vi "Multichannel Recording0.1.vi"() -> ()   [LabVIEW 2014]
uses:
  Timed Recorder Project/Single Channel Volt Recording Folder/Enum State Typedef.ctl
  <vilib>/Utility/error.llb/DialogType.ctl
  <vilib>/_DAQmxBase/Internals/DAQmxBase Create Channel (AI-Voltage-Basic).vi
  <vilib>/_DAQmxBase/Internals/DAQmxBase Timing (Sample Clock).vi
  <vilib>/_DAQmxBase/Internals/DAQmxBase Read (Analog 2D DBL NChan NSamp).vi
panel:
  in  "Tab Control":T1(tab)
  in  "Use Channel 0":bool caption="In Use?"
  in  "Amplifier Channel 0":T2 {"Amplifier Model" items=["Select a Model", "AM 1700", "BMA 200"]}
  out "Channel 0 Chart":waveform(dbl)(graph)
  in  "User Data Channel 0":T3
  in  "Use Channel 1":bool caption="In Use?"
  out "Channel 1 Chart":waveform(dbl)(graph)
  in  "User Data Channel 1":T3
  in  "Amplifier Channel 1":T2 {"Amplifier Model" items=["Select a Model", "AM 1700", "BMA 200"]}
  in  "Use Channel 2":bool caption="In Use?"
  out "Channel 2 Chart":waveform(dbl)(graph)
  in  "User Data Channel 2":T3
  in  "Amplifier Channel 2":T2 {"Amplifier Model" items=["Select a Model", "AM 1700", "BMA 200"]}
  in  "Use Channel 3":bool caption="In Use?"
  out "Channel 3 Chart":waveform(dbl)(graph)
  in  "User Data Channel 3":T3
  in  "Amplifier Channel 3":T2 {"Amplifier Model" items=["Select a Model", "AM 1700", "BMA 200"]}
  out "Overview Chart":waveform(dbl)[](graph)
  in  "Stop Preview":bool
  in  "OK Button":bool
  out "State":T4
  in  "Clear Display":bool
  in  "Preview Button":bool
  out "Iterations Recorded":i32
  in  "Recording Time (seconds)":dbl
  in  "Sample Rate":i32=1000
  in  "Stop Button":bool
  out "Start Time hr/min":string
  out "Date mm/dd/yy":string
  in  "Exit Button":bool
  in  "Record Button":bool
  # "MSU EFISH Lab Single Channel Electronic Pulse Recorder"
  # "Must enter numbers into here before you start"
  # "Blue for On\nOrange for Off"
  # "DC"
  # "AC"
  # "Blue for AC and Orange for DC"
  # "Blue for On\nOrange for Off"
  # "DC"
  # "AC"
  # "Blue for AC and Orange for DC"
  # "Blue for On\nOrange for Off"
  # "DC"
  # "AC"
  # "Blue for AC and Orange for DC"
  # "Blue for On\nOrange for Off"
  # "DC"
  # "AC"
  # "Blue for AC and Orange for DC"
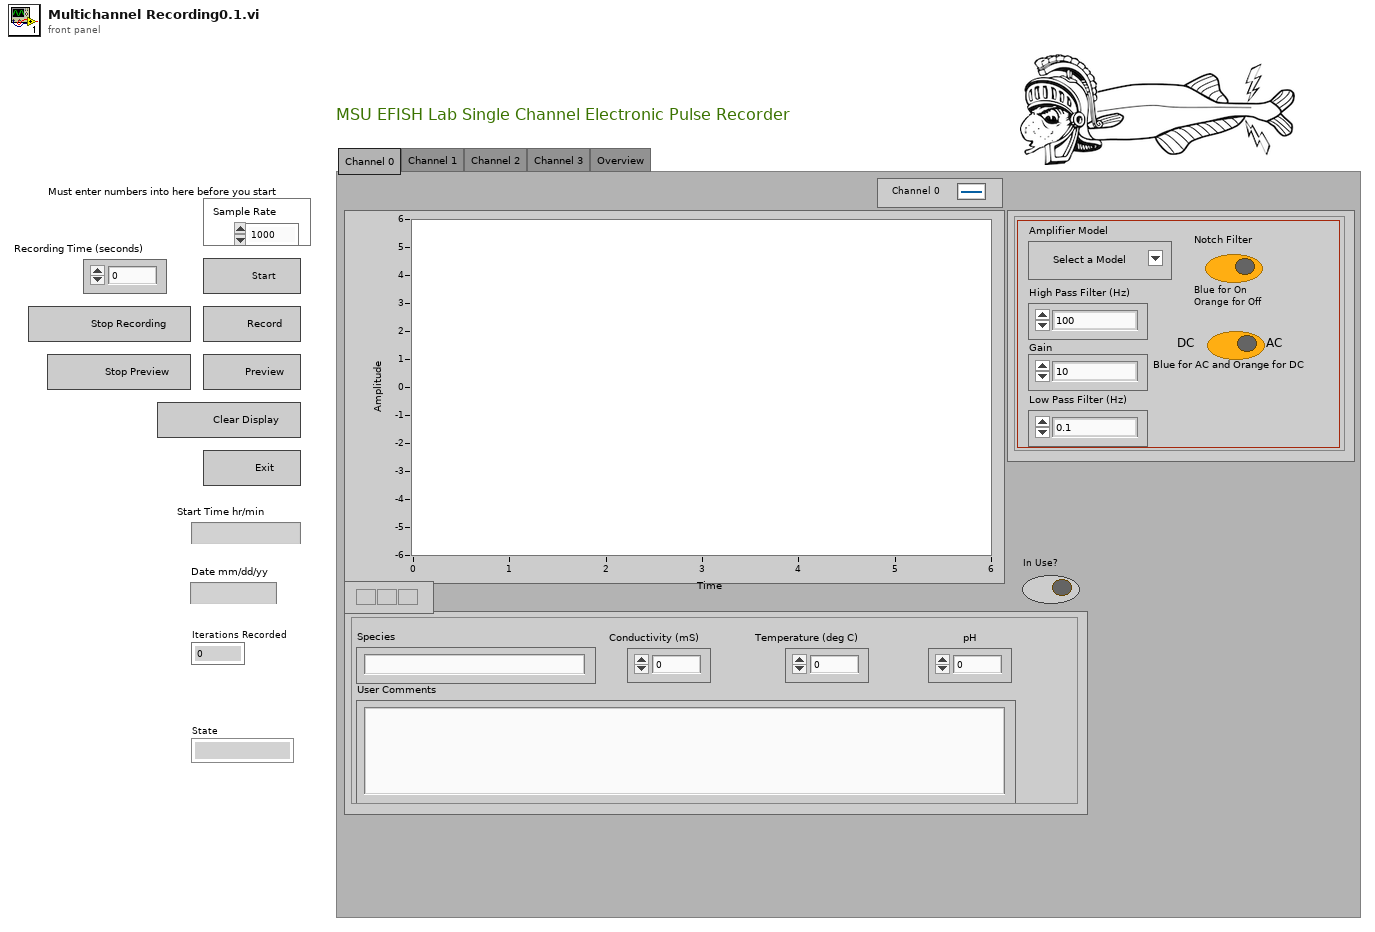
[diagram p1: front panel]
types:
  T1 = enum32{"Channel 0", "Channel 1", "Channel 2", "Channel 3", "Overview"}
  T2 = cluster{"Low Pass Filter (Hz)":enum16{"0.1", "1", "3", "10", "30", "100", "300"}, "Gain ":enum16{"10", "20", "50", "100", "200", "500", "1000", "2k", "5k", "10k", "20k", "50k"}, "High Pass Filter (Hz)":enum16{"100", "500", "1000", "3000", "5000", "10,000", "20,000", "30,000", "50,000"}, "Notch Filter":bool, "Amplifier Model":u16, "AC/DC Switch":bool}
  T3 = cluster{"pH":dbl, "Conductivity (mS)":dbl, "Temperature (deg C)":dbl, "User Comments":string, "Species":string}
  T4 = typedef "Enum State Typedef.ctl" = enum16{"", "Beginning State", "Set the Sample Clock", "Prepreview Handling", "Clear Display", "Preview Data", "Stop", "Exit", "Record", "Create File"}
  T5 = enum16{"open", "open or create", "create or replace", "create", "open (read-only)"}
  T6 = typedef "DialogType.ctl" = u16
  T7 = cluster{"data":dbl[][], dbl[][], i32, i32, dbl, "Use Channel 2":bool}
  T8 = cluster{"data":dbl[][], dbl[][], i32, i32, dbl, "Use Channel 1":bool}
  T9 = cluster{"data":dbl[][], dbl[][], i32, i32, dbl, "Use Channel 0":bool}
  T10 = cluster{"data":dbl[][], dbl[][], i32, i32, dbl, "Use Channel 3":bool}
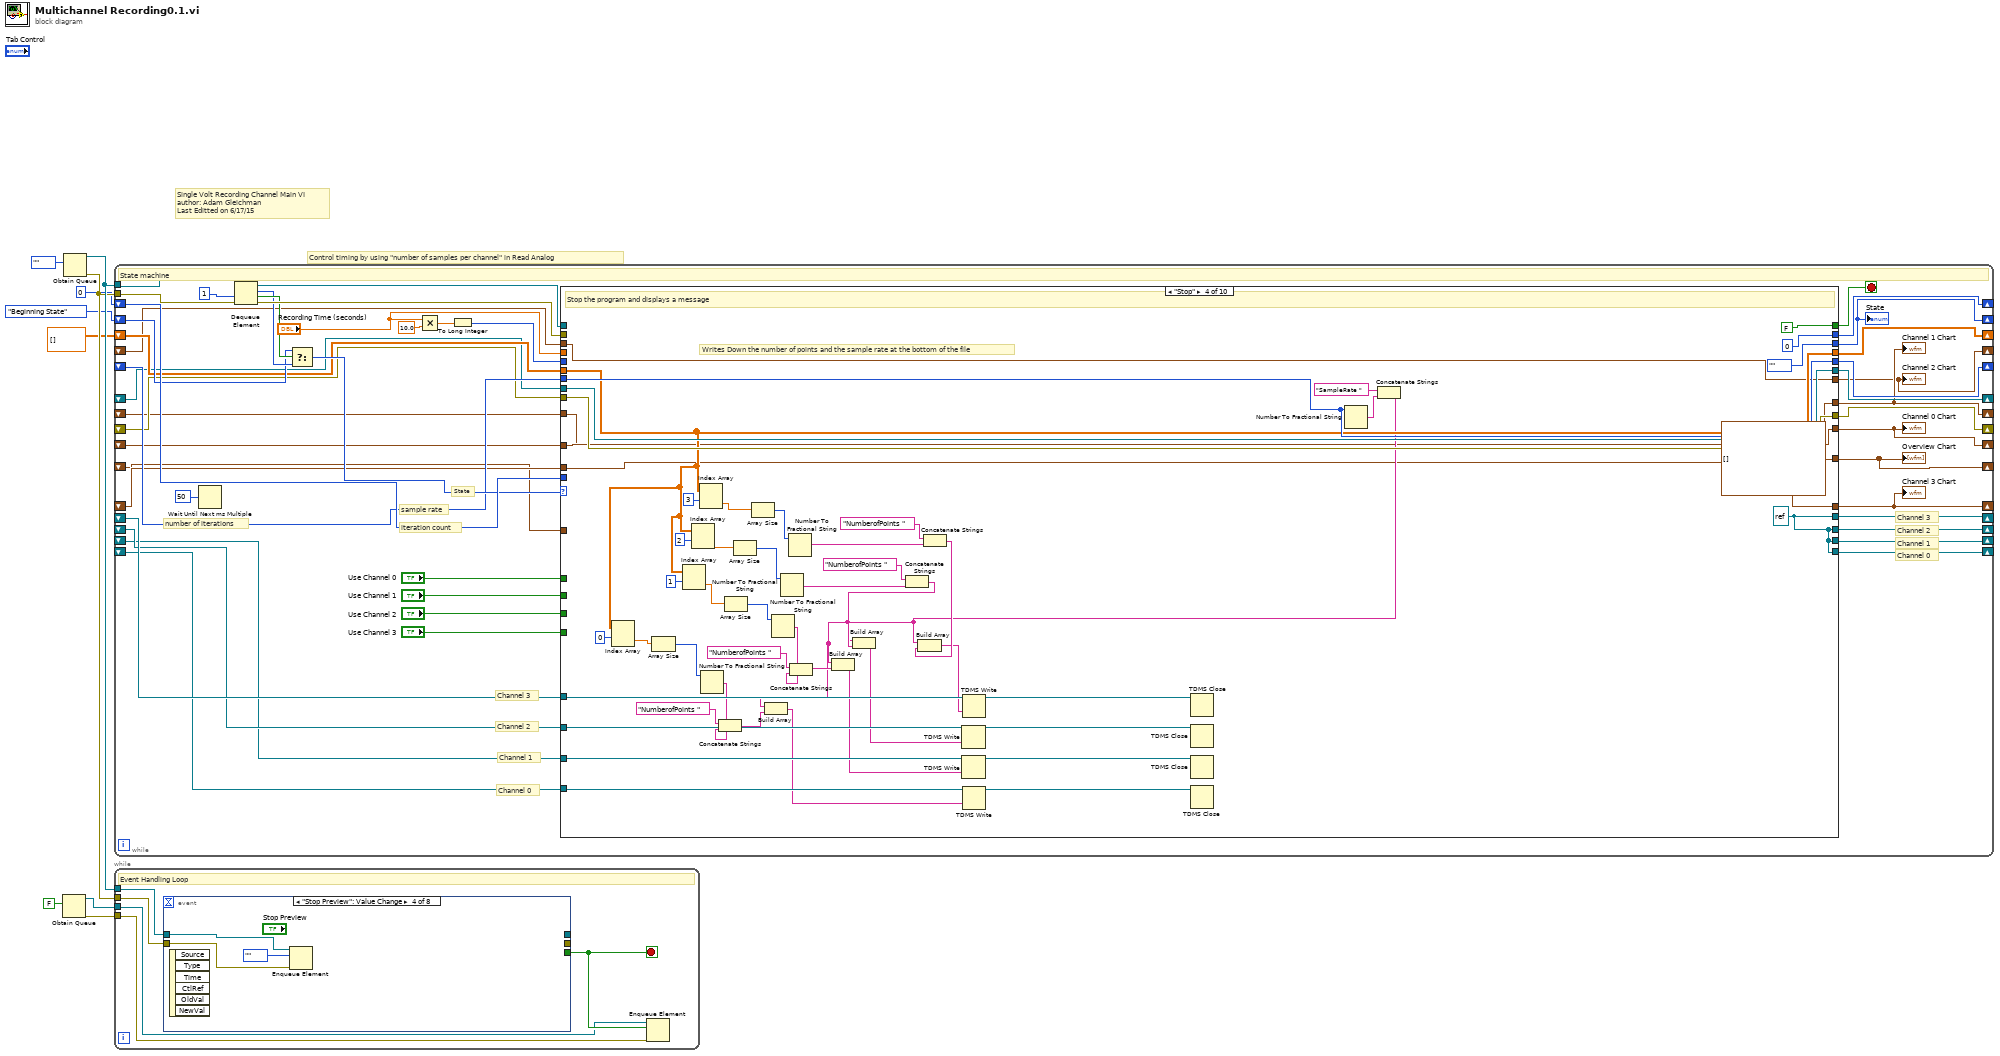
[diagram p0: block diagram]
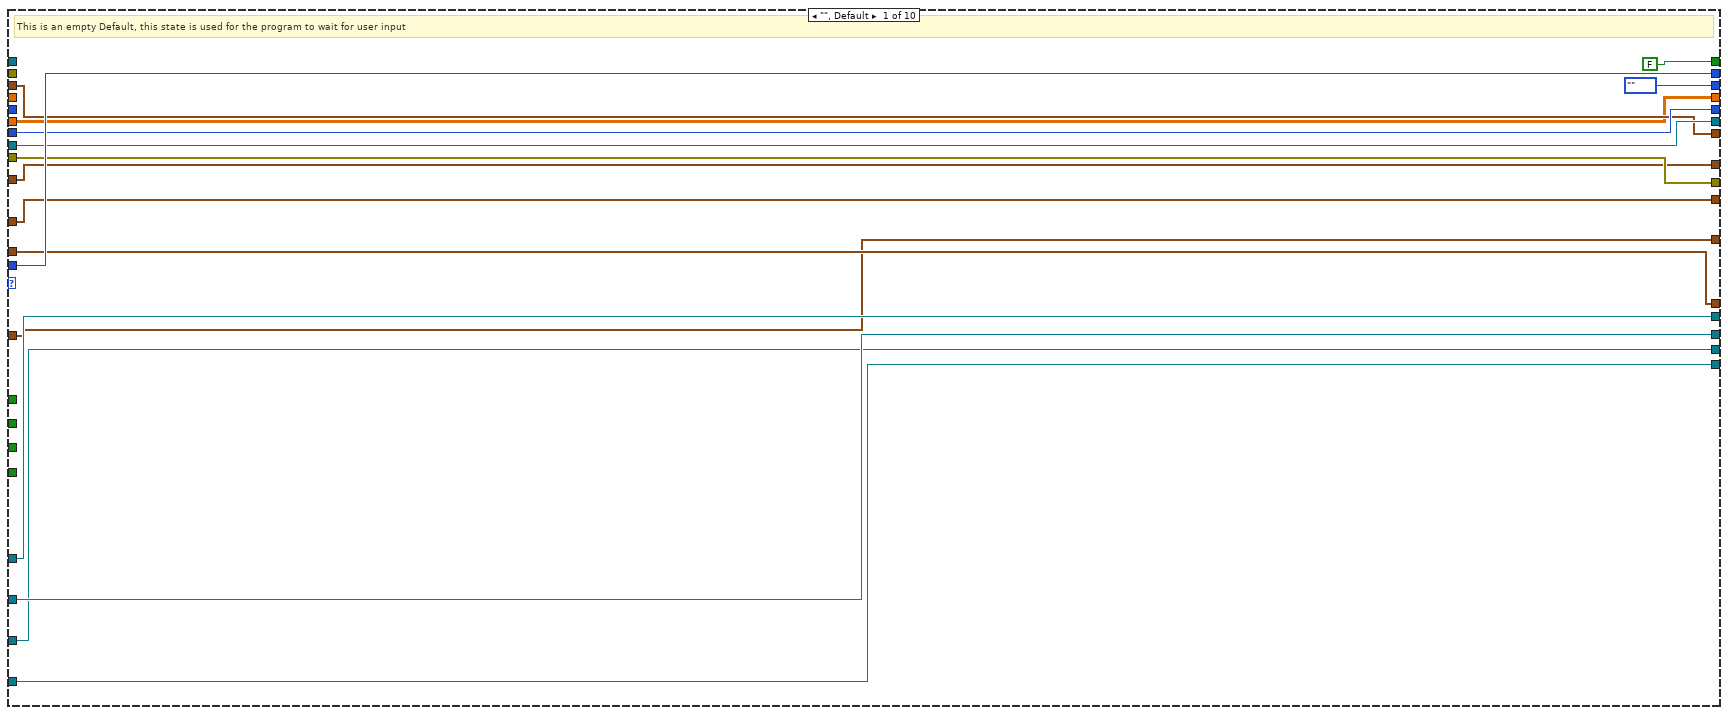
[diagram p2: hidden frame]
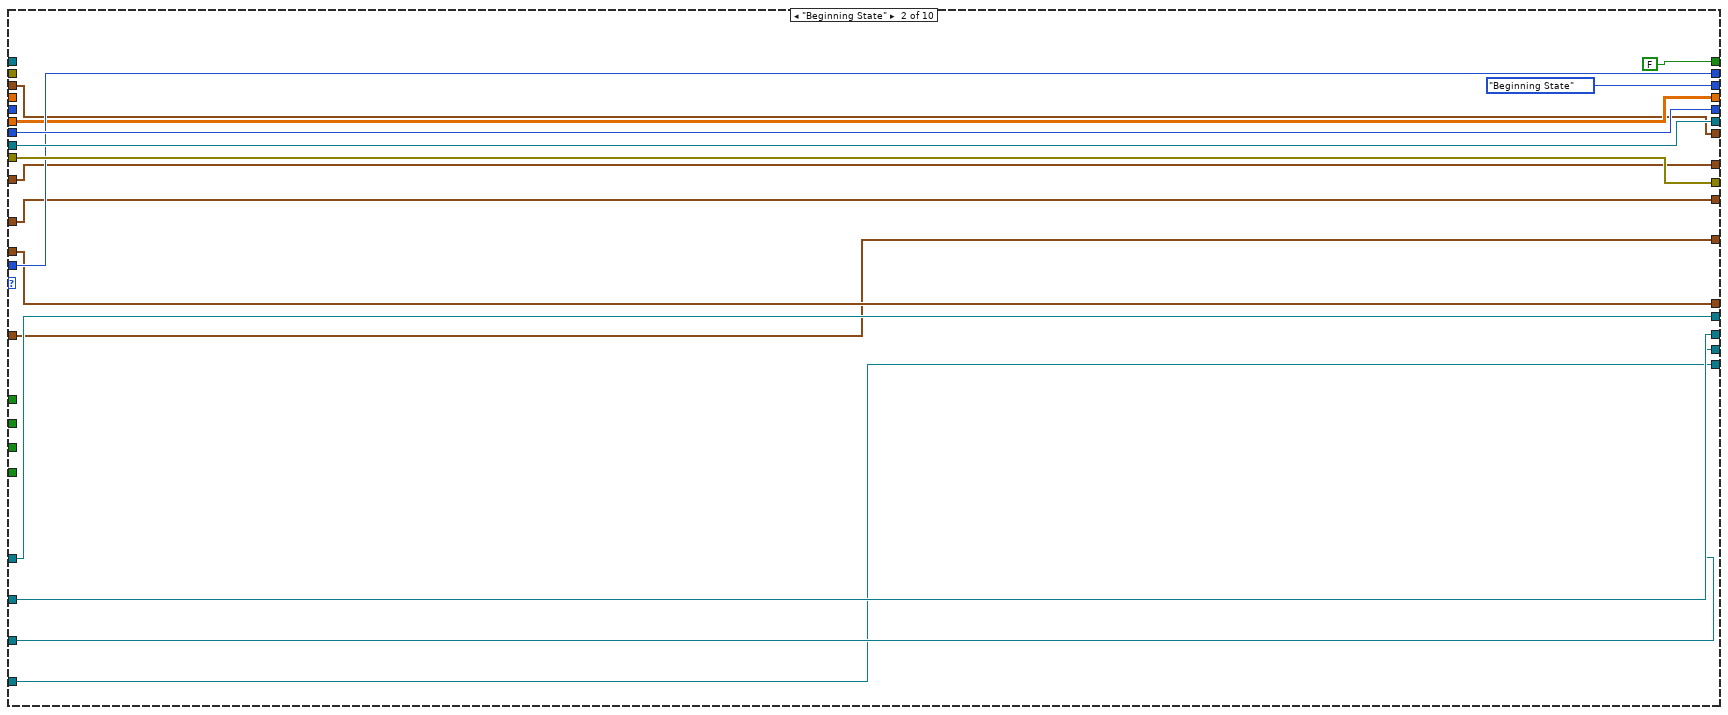
[diagram p3: hidden frame]
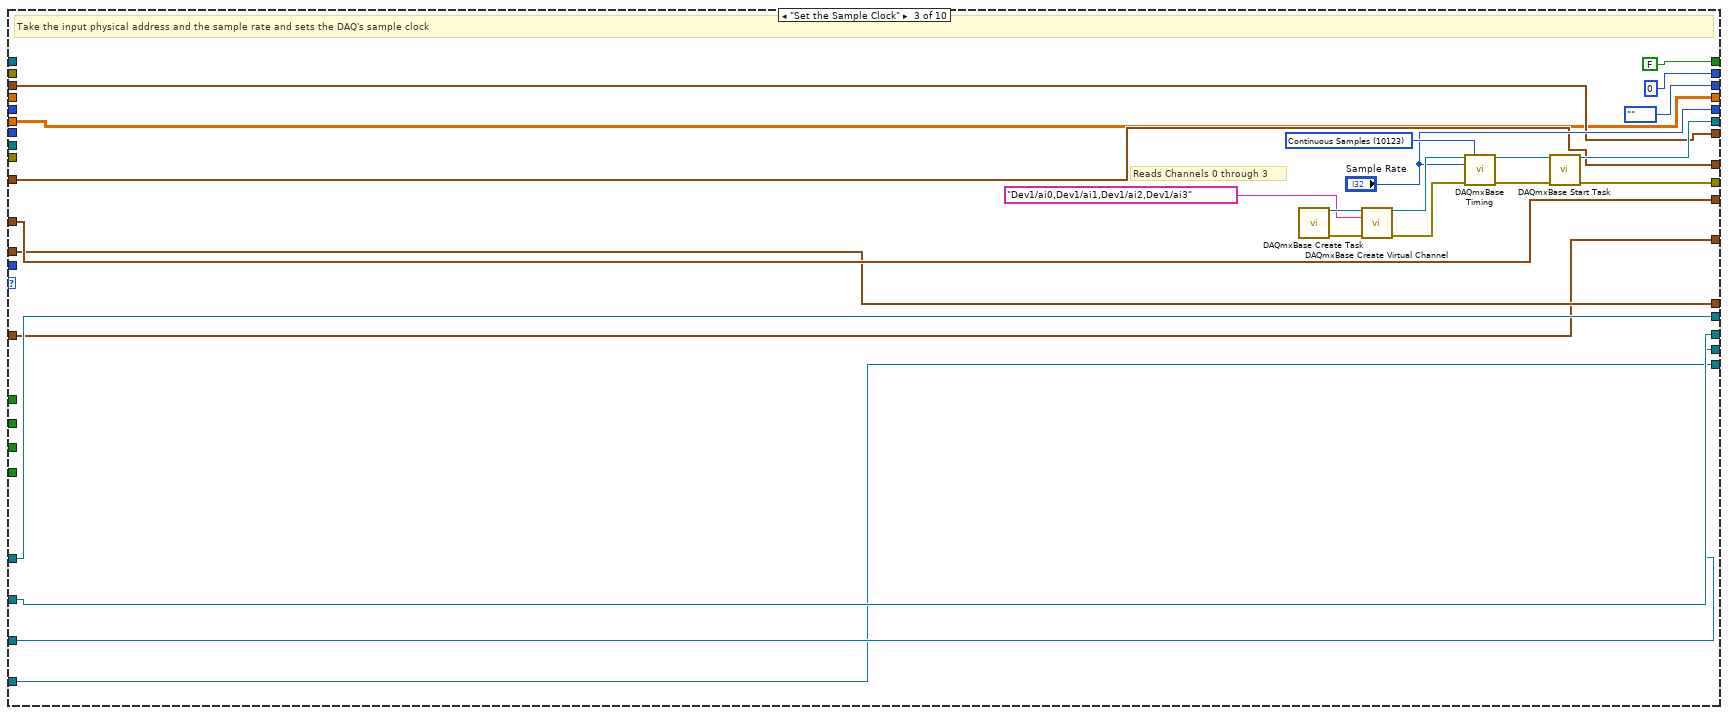
[diagram p4: hidden frame]
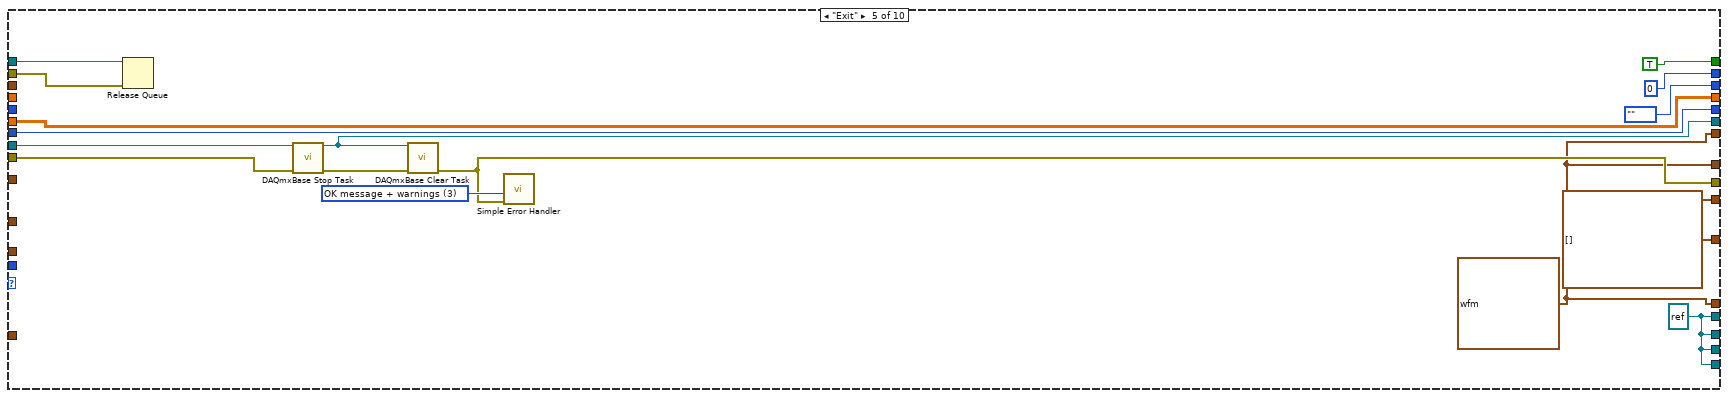
[diagram p5: hidden frame]
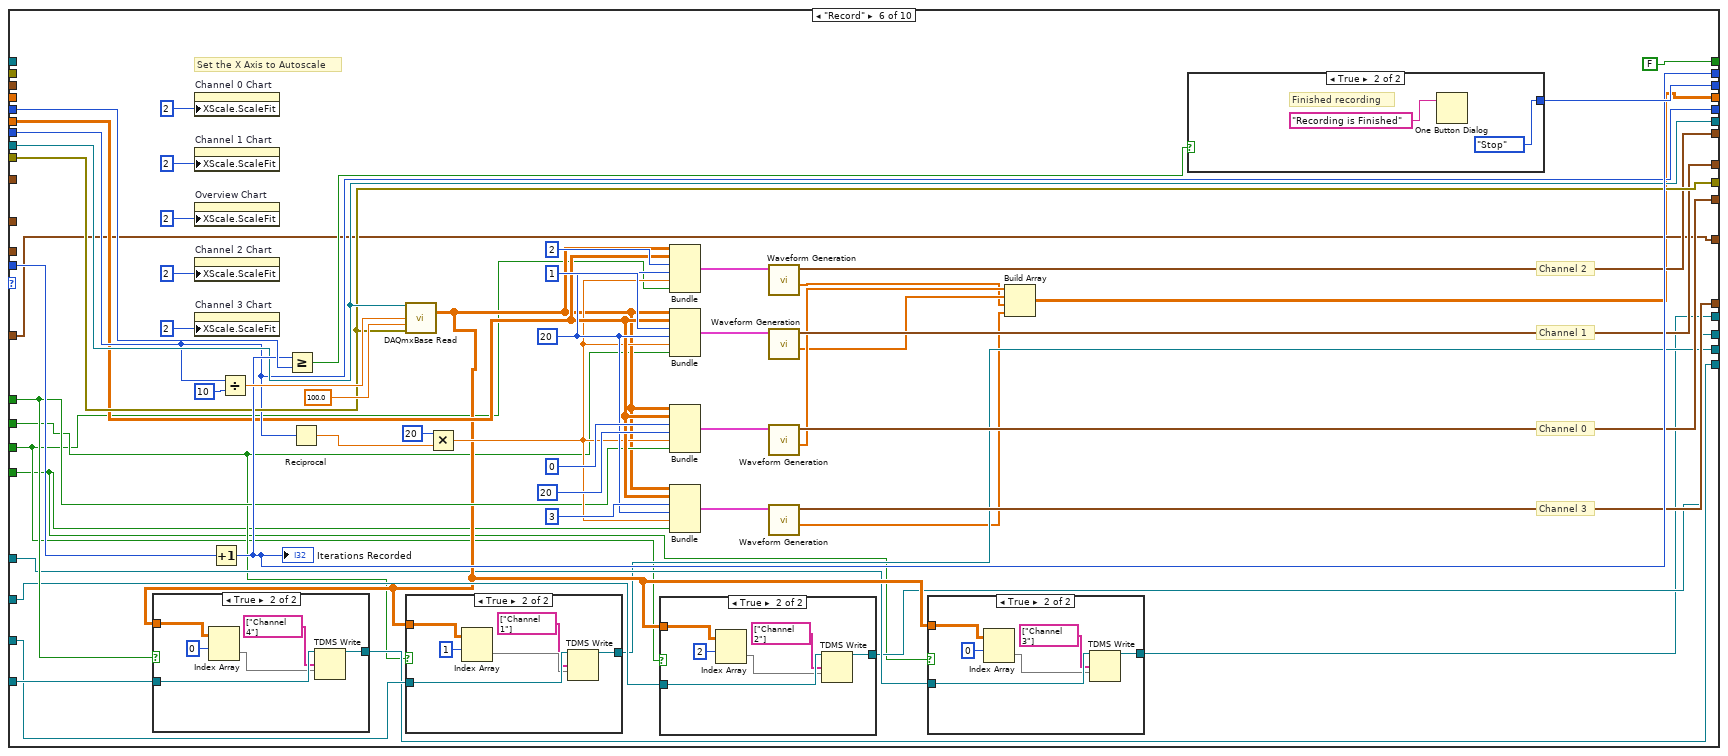
[diagram p6: hidden frame]
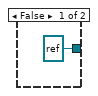
[diagram p7: hidden frame]
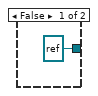
[diagram p8: hidden frame]
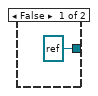
[diagram p9: hidden frame]
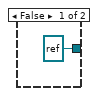
[diagram p10: hidden frame]
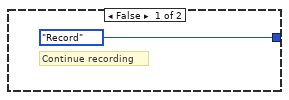
[diagram p11: hidden frame]
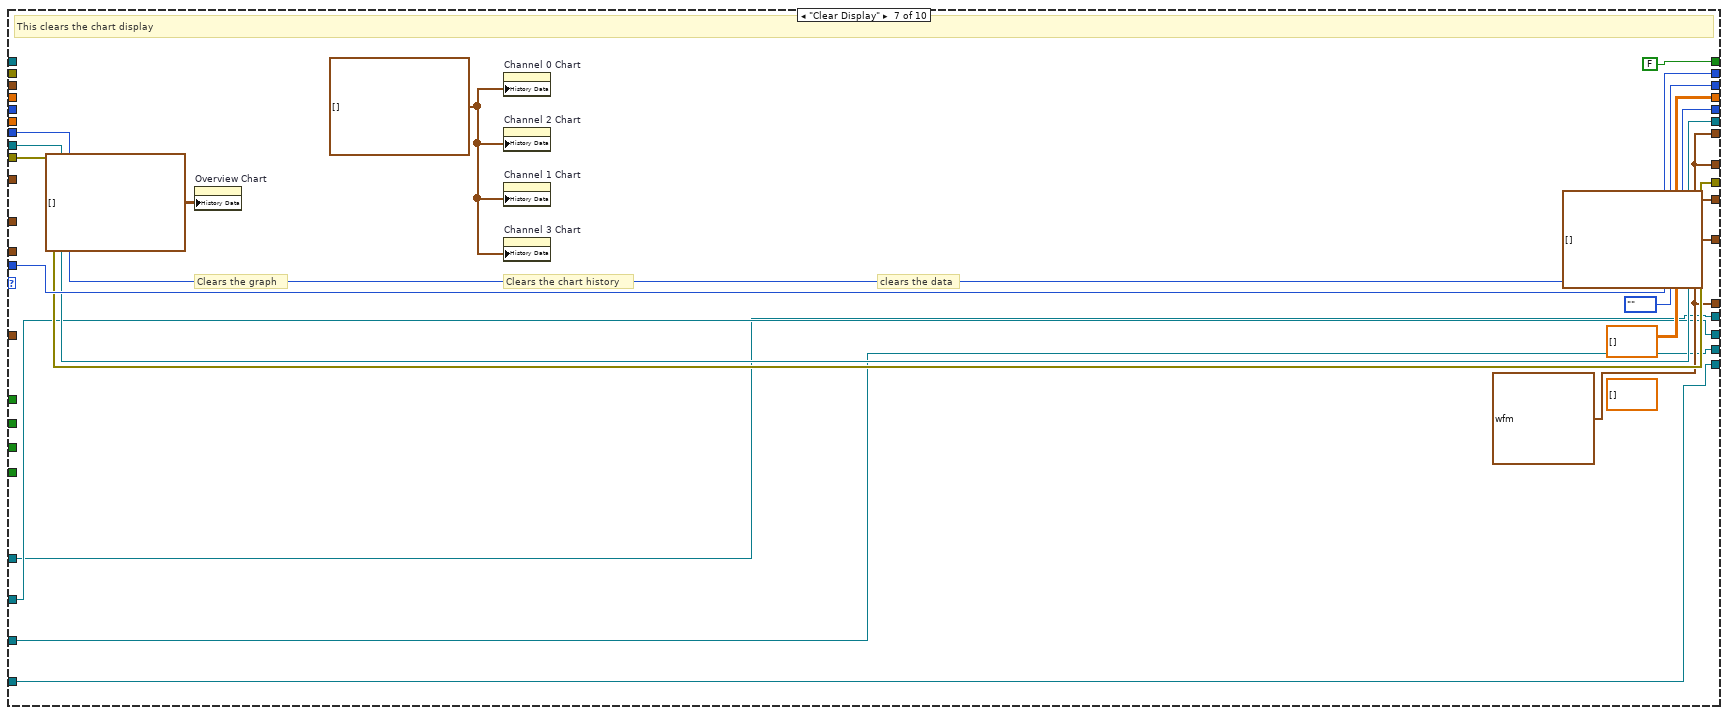
[diagram p12: hidden frame]
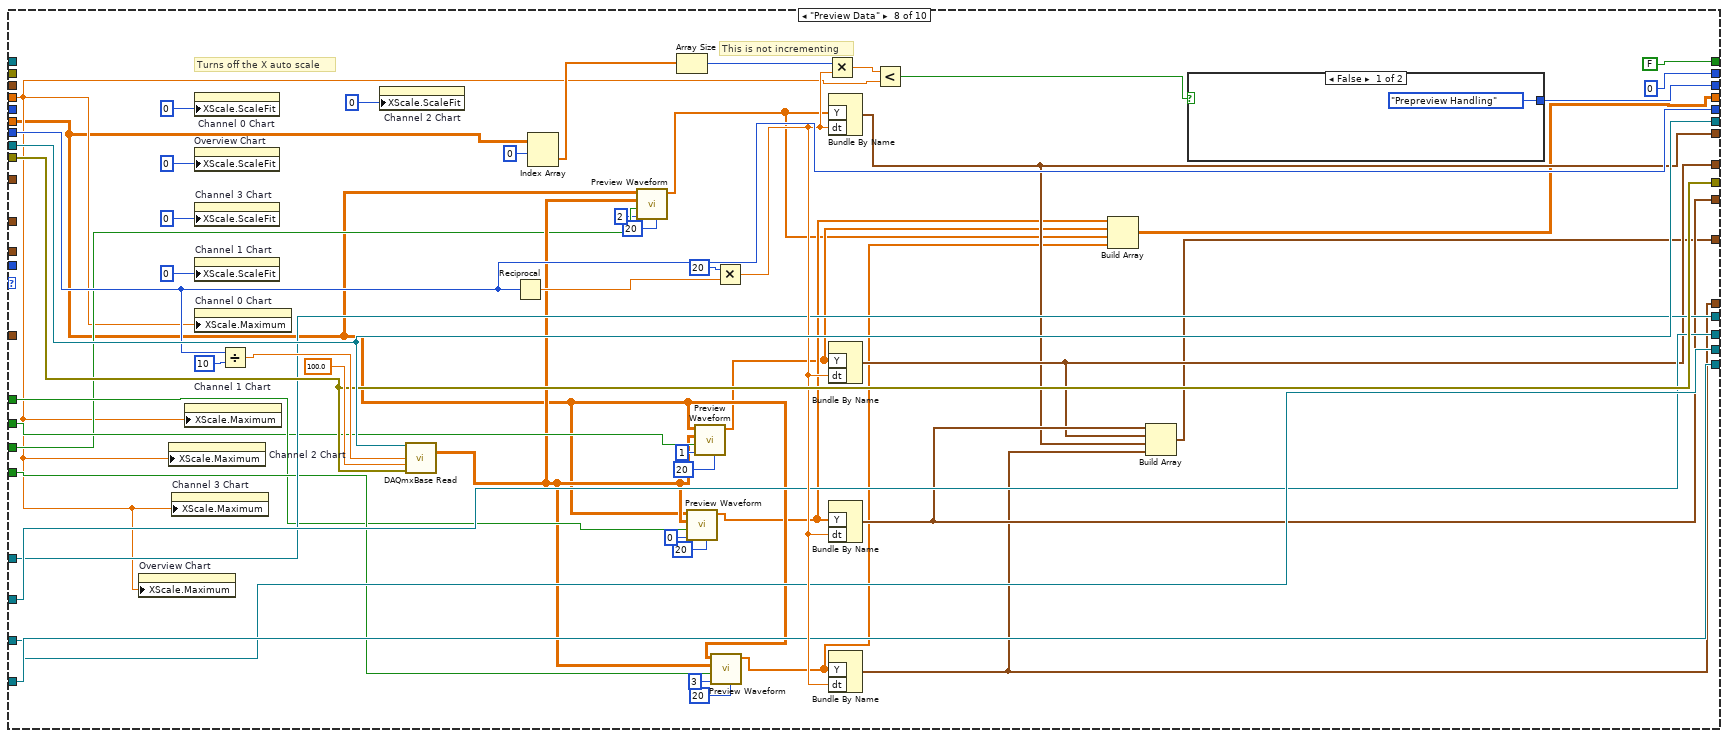
[diagram p13: hidden frame]
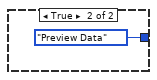
[diagram p14: hidden frame]
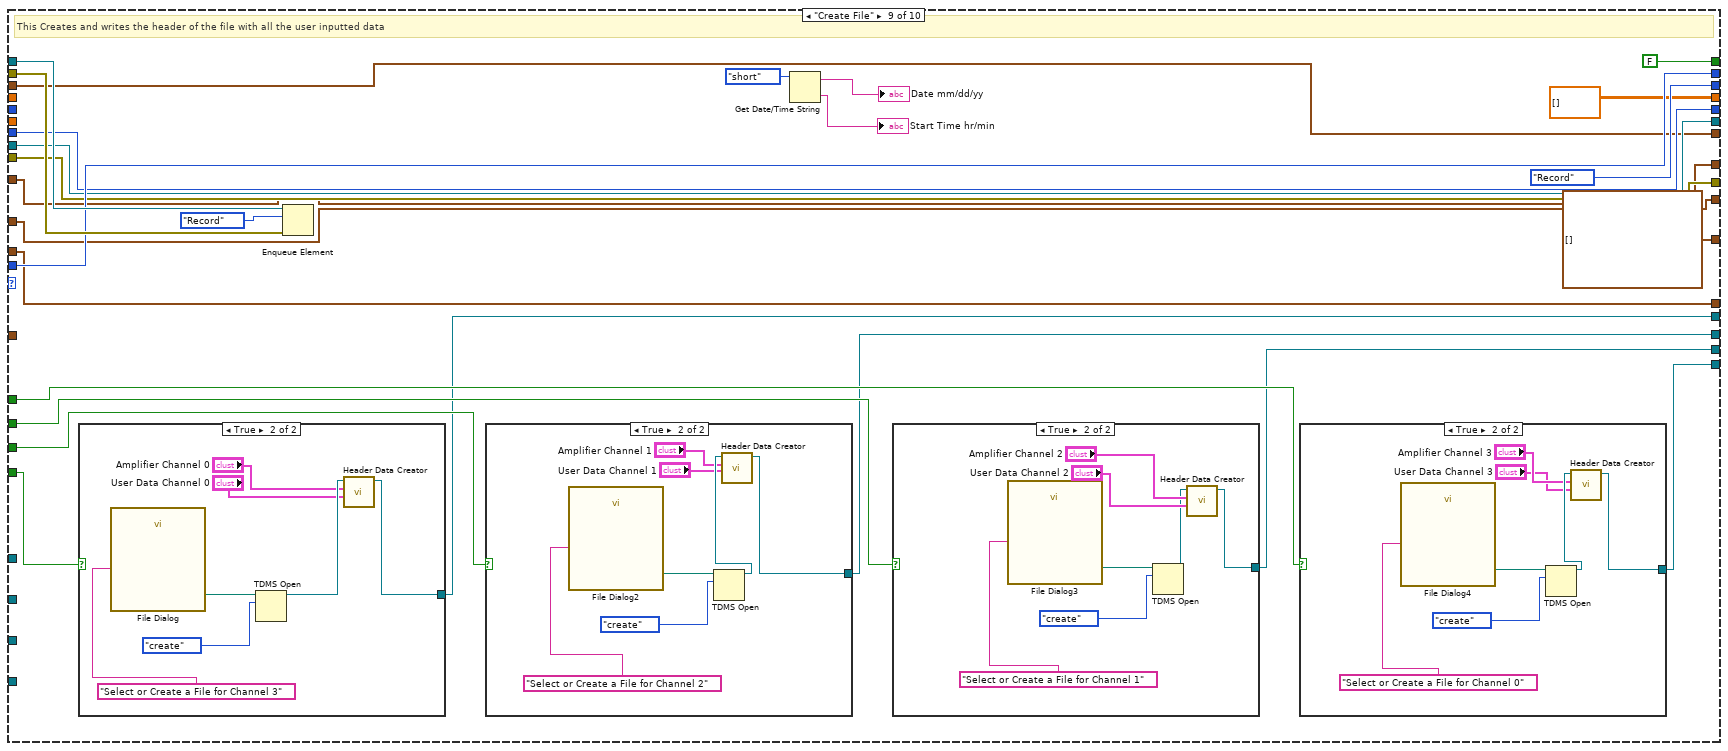
[diagram p15: hidden frame]
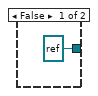
[diagram p16: hidden frame]
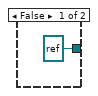
[diagram p17: hidden frame]
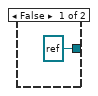
[diagram p18: hidden frame]
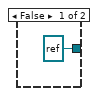
[diagram p19: hidden frame]
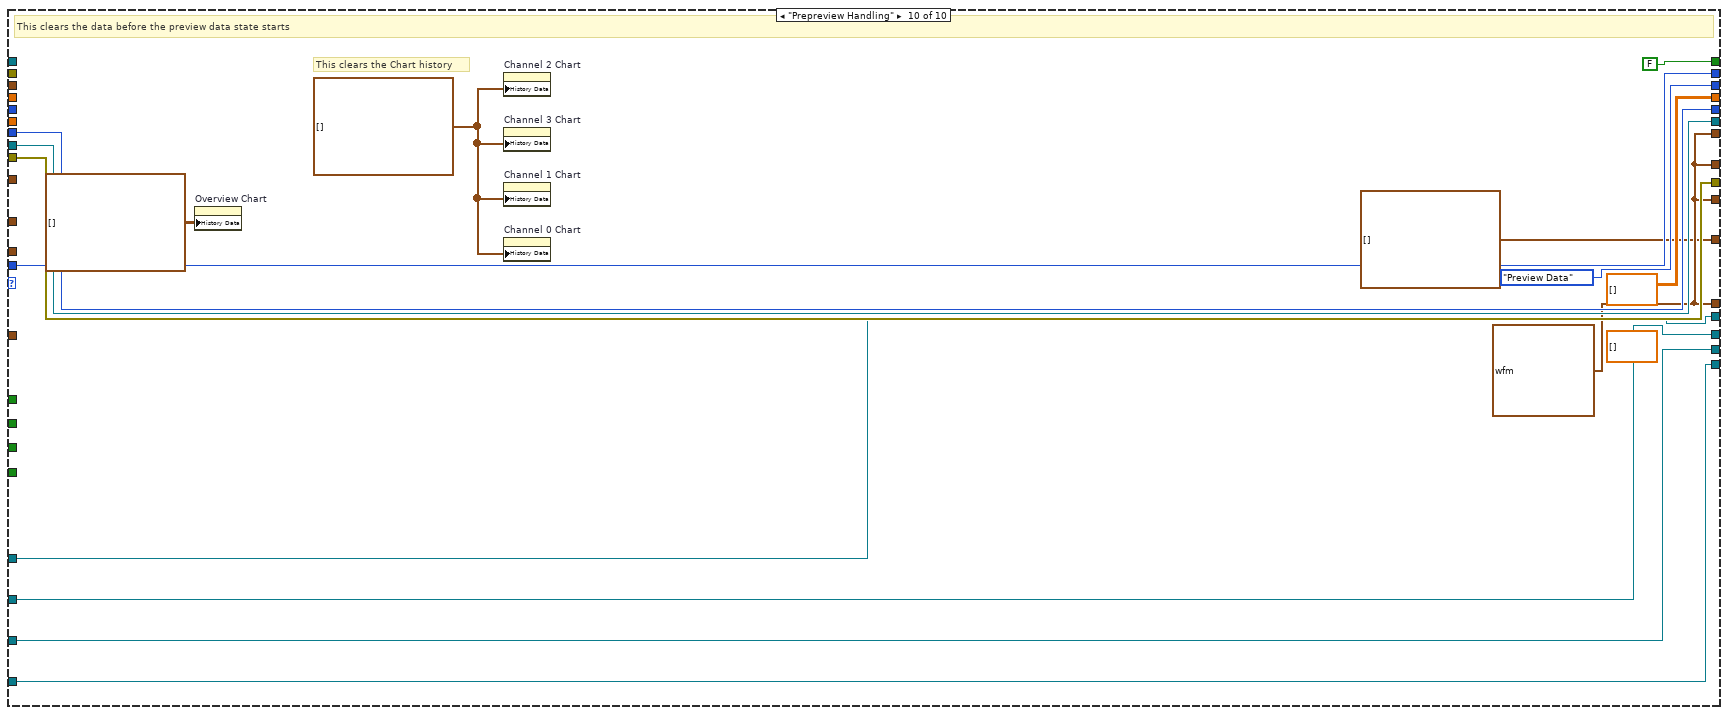
[diagram p20: hidden frame]
diagram:
  # "Single Volt Recording Channel Main VI\nauthor: Adam Gleichman\nLast Editted on 6/17/15"
  # "Control timing by using \"number of samples per channel\" in Read Analog"
  n1 = Obtain Queue(element data type=FALSE) -> (queue out=w2:refnum<queue>, error out=w1:errorcluster)  [unwired: 4 in, 1 out]
  n2 = Obtain Queue(element data type=Enum_State_Typedef."" ("State")) -> (queue out=w8:refnum<queue>, error out=w7:errorcluster)  [unwired: 4 in, 1 out]
  n3 = while {
    tunnel: w8 -> [w57]
    tunnel: w7 -> [w56]
    shift-right: [w49] -> _
    shift-left: 0 -> [w50]
    shift-right: [w44] -> _
    shift-left: Enum_State_Typedef."Beginning State" ("State") -> [w46]
    shift-right: [w42] -> _
    shift-left: _ -> [w43]
    shift-right: [w37] -> _
    shift-left: dbl[][] [] -> [w39]
    shift-right: [w27] -> _
    shift-left: _ -> [w38]
    shift-right: [w35] -> _
    shift-left: _ -> [w33]
    shift-right: [w34] -> _
    shift-left: _ -> [w32]
    shift-right: [w29] -> _
    shift-left: _ -> [w12]
    shift-right: [w28] -> _
    shift-left: _ -> [w14]
    shift-right: [w30] -> _
    shift-left: _ -> [w13]
    shift-right: [w22] -> _
    shift-left: _ -> [w18]
    shift-right: [w21] -> _
    shift-left: _ -> [w17]
    shift-right: [w19] -> _
    shift-left: _ -> [w16]
    shift-right: [w20] -> _
    shift-left: _ -> [w15]
    shift-right: [w11] -> _
    shift-left: _ -> [w10]
    stop <- w55 stop-if-true
    # "Channel 0"
    # "Channel 1"
    # "Channel 2"
    # "Channel 3"
    # "Channel 0"
    # "Channel 1"
    # "Channel 2"
    # "Channel 3"
    # "State"
    # "iteration count"
    # "sample rate"
    # "number of iterations"
    # "State machine"
    n4 = Wait Until Next ms Multiple(millisecond multiple=u32 50) -> ()  [unwired: 1 out]
    n5 = Dequeue Element(queue=w57, timeout in ms (-1)=1, error in (no error)=w56) -> (queue out=w54:refnum<queue>, element=w47:T4, timed out?=w48:bool, error out=w53:errorcluster)
    n6 = Select(t=w46, s=w48, f=w47) -> (s? t:f=w45:T4)
    n7 = Multiply(x="Recording Time (seconds)", y=10.0) -> (x*y=w31:dbl)
    n8 = To Long Integer(number=w31) -> (32bit integer=w51:i32)
    n9 = case shown="\"Stop\"" w45 {
      tunnel: [FALSE FALSE FALSE FALSE TRUE FALSE FALSE FALSE FALSE FALSE] -> w55
      tunnel: w54 -> [_ _ _ _ w176 _ _ _ w360 _]
      tunnel: w53 -> [_ _ _ _ w175 _ _ _ w359 _]
      tunnel: w33 -> [w69 w87 _ w162 w179 w224 w278 w321 w353 w403]
      tunnel: w32 -> [w68 w88 _ w161 w178 w223 w277 w320 w352 w402]
      tunnel: w43 -> [w70 w85 _ w159 w172 w222 w276 w317 w356 w404]
      tunnel: w51 -> [_ _ _ _ _ w232 _ _ _ _]
      tunnel: w50 -> [w72 w84 _ _ _ w233 w281 _ w357 w405]
      tunnel: [w72 w84 0 ("Sample Rate") 0 0 w227 w281 0 w357 w405] -> w49
      tunnel: [Enum_State_Typedef."" ("State") Enum_State_Typedef."Beginning State" ("State") Enum_State_Typedef."" ("State") Enum_State_Typedef."" ("State") Enum_State_Typedef."" ("State") w229 Enum_State_Typedef."" ("State") w325 Enum_State_Typedef."Record" ("State") Enum_State_Typedef."Preview Data" ("State")] -> w44
      tunnel: [w70 w85 "Sample Rate" w159 w172 w222 w276 w317 w356 w404] -> w42
      tunnel: [w59 w79 w95 w130 w171 w182 dbl[][] [] w282 dbl[][] [] dbl[][] []] -> w37
      tunnel: w39 -> [w59 w79 w95 w130 w171 w202 _ w292 _ _]
      tunnel: w38 -> [w63 w78 w99 w123 _ _ _ _ w339 _]
      tunnel: "Recording Time (seconds)" -> [_ _ _ _ _ _ _ w293 _ _]
      tunnel: [w69 w87 w106 w162 w170 w224 w278 w321 w353 w403] -> w35
      tunnel: [w68 w88 w105 w161 w169 w223 w277 w320 w352 w402] -> w34
      tunnel: [w63 w78 w99 w123 w167 w207 w273 w289 w339 w400] -> w27
      tunnel: [w62 w77 w98 w124 w167 w206 w273 w290 w338 w400] -> w28
      tunnel: [w60 w75 w96 w126 w167 w205 w273 w288 w336 w400] -> w29
      tunnel: [w61 w76 w97 w125 w167 w204 w273 w291 w337 w400] -> w30
      tunnel: "Use Channel 2" -> [_ _ _ _ _ w189 _ w296 w350 _]
      tunnel: "Use Channel 1" -> [_ _ _ _ _ w190 _ w299 w349 _]
      tunnel: "Use Channel 0" -> [_ _ _ _ _ w200 _ w303 w348 _]
      tunnel: "Use Channel 3" -> [_ _ _ _ _ w188 _ w306 w351 _]
      tunnel: [w67 w83 w94 w157 w168 w191 w269 w308 w343 w395] -> w22
      tunnel: [w66 w82 w93 w157 w168 w192 w270 w309 w342 w396] -> w21
      tunnel: [w65 w81 w92 w157 w168 w193 w271 w310 w341 w397] -> w19
      tunnel: [w64 w80 w91 w157 w168 w194 w272 w311 w340 w398] -> w20
      tunnel: w18 -> [w67 w83 w94 w153 _ w195 w269 w308 _ w395]
      tunnel: w17 -> [w66 w82 w93 w149 _ w197 w270 w309 _ w396]
      tunnel: w16 -> [w65 w81 w92 w142 _ w198 w271 w310 _ w397]
      tunnel: w15 -> [w64 w80 w91 w140 _ w199 w272 w311 _ w398]
      tunnel: w14 -> [w62 w77 w98 w124 _ _ _ _ w338 _]
      tunnel: w13 -> [w61 w76 w97 w125 _ _ _ _ w337 _]
      tunnel: w12 -> [w60 w75 w96 w126 _ _ _ _ w336 _]
      tunnel: [w58 w74 w90 waveform(dbl)[] [] waveform(dbl)[] [] w187 waveform(dbl)[] [] w287 waveform(dbl)[] [] waveform(dbl)[] []] -> w11
      tunnel: w10 -> [w58 w74 w90 _ _ w187 _ _ _ _]
      frame "", Default {
        # "This is an empty Default, this state is used for the program to wait for user input"
      }
      frame "Beginning State" {
      }
      frame "Set the Sample Clock" {
        w109 = 10123 items=["Finite Samples"=10178, "Continuous Samples"=10123, "Hardware Timed Single Point"=12522] ("sample mode")
        # "Reads Channels 0 through 3"
        # "Take the input physical address and the sample rate and sets the DAQ's sample clock"
        n10 = call <vilib>:"DAQmxBase Create Task.vi"() -> ("task out"=w113:refnum<k21>, "error out"=w112:errorcluster)  [unwired: 14 in]
        n11 = call-poly <vilib>:"DAQmxBase Create Virtual Channel.vi"("task in"=w113, "physical channels"=tag "Dev1/ai0,Dev1/ai1,Dev1/ai2,Dev1/ai3", "error in"=w112) -> ("task out"=w111:refnum<k21>, "error out"=w110:errorcluster)  [unwired: 11 in]
        n12 = call-poly <vilib>:"DAQmxBase Timing.vi"("task/channels in"=w111, "sample mode"=w109, "rate"="Sample Rate", "error in"=w110) -> ("task out"=w108:refnum<k21>, "error out"=w107:errorcluster)  [unwired: 10 in]
        n13 = call <vilib>:"DAQmxBase Start Task.vi"("task/channels in"=w108, "error in"=w107) -> ("task out"=w106:refnum<k21>, "error out"=w105:errorcluster)  [unwired: 12 in]
      }
      frame "Stop" {
        w157 = refnum<k34> refnum ("tdms file out")
        # "Writes Down the number of points and the sample rate at the bottom of the file"
        # "Stop the program and displays a message"
        n14 = Index Array(array=w130, index (row)=0) -> (element=w115:dbl[])  [unwired: 1 in]
        n15 = Array Size(array=w115) -> (size(s)=w114:i32)
        n16 = Index Array(array=w130, index (row)=1) -> (element=w117:dbl[])  [unwired: 1 in]
        n17 = Index Array(array=w130, index (row)=2) -> (element=w119:dbl[])  [unwired: 1 in]
        n18 = Index Array(array=w130, index (row)=3) -> (element=w121:dbl[])  [unwired: 1 in]
        n19 = Number To Fractional String(number=w114) -> (F-format string=w131:string)  [unwired: 3 in]
        n20 = Concatenate Strings("NumberofPoints " ("string"), w131) -> (w128:string)
        n21 = Array Size(array=w117) -> (size(s)=w116:i32)
        n22 = Array Size(array=w119) -> (size(s)=w118:i32)
        n23 = Array Size(array=w121) -> (size(s)=w120:i32)
        n24 = Number To Fractional String(number=w116) -> (F-format string=w136:string)  [unwired: 3 in]
        n25 = Number To Fractional String(number=w118) -> (F-format string=w145:string)  [unwired: 3 in]
        n26 = Number To Fractional String(number=w120) -> (F-format string=w154:string)  [unwired: 3 in]
        n27 = Concatenate Strings("NumberofPoints " ("string"), w136) -> (w135:string)
        n28 = Concatenate Strings("NumberofPoints " ("string"), w145) -> (w144:string)
        n29 = Concatenate Strings("NumberofPoints " ("string"), w154) -> (w151:string)
        n30 = Number To Fractional String(number=w159) -> (F-format string=w158:string)  [unwired: 3 in]
        n31 = Concatenate Strings("SampleRate ", w158) -> (w129:string)
        n32 = Build Array(w129, w128) -> (w127:string[])
        n33 = Build Array(w129, w135) -> (w134:string[])
        n34 = Build Array(w129, w144) -> (w143:string[])
        n35 = Build Array(w129, w151) -> (w150:string[])
        n36 = TDMS Write(0:w149, 9:w143) -> (4:w148:refnum<k34>)  [unwired: 4 in, 3 out]
        n37 = TDMS Write(0:w142, 9:w134) -> (4:w141:refnum<k34>)  [unwired: 4 in, 3 out]
        n38 = TDMS Write(0:w153, 9:w150) -> (4:w152:refnum<k34>)  [unwired: 4 in, 3 out]
        n39 = TDMS Write(0:w140, 9:w127) -> (4:w139:refnum<k34>)  [unwired: 4 in, 3 out]
        n40 = TDMS Close(11:w152) -> ()  [unwired: 1 in, 2 out]
        n41 = TDMS Close(11:w148) -> ()  [unwired: 1 in, 2 out]
        n42 = TDMS Close(11:w141) -> ()  [unwired: 1 in, 2 out]
        n43 = TDMS Close(11:w139) -> ()  [unwired: 1 in, 2 out]
      }
      frame "Exit" {
        w167 = waveform(dbl) {"t0"=timestamp(0 s since 1904-01-01), "dt"=1.0, "Y"=[]} ("Waveform")
        w168 = refnum<k34> refnum ("tdms file out")
        w177 = T6 3 items=["no dialog", "OK message", "continue or stop message", "OK message + warnings", "continue/stop + warnings"] ("type of dialog (OK msg:1)")
        n44 = Release Queue(queue=w176, error in (no error)=w175) -> ()  [unwired: 1 in, 3 out]
        n45 = call <vilib>:"DAQmxBase Stop Task.vi"("task/channels in"=w179, "error in"=w178) -> ("task out"=w170:refnum<k21>, "error out"=w180:errorcluster)  [unwired: 12 in]
        n46 = call <vilib>:"DAQmxBase Clear Task.vi"("task in"=w170, "error in"=w180) -> ("error out"=w169:errorcluster)  [unwired: 13 in]
        n47 = call <vilib>:"Simple Error Handler.vi"("type of dialog (OK msg:1)"=w177, "error in (no error)"=w169) -> ()  [unwired: 3 in, 5 out]
      }
      frame "Record" {
        w213 = 20
        # "Channel 1"
        # "Channel 2"
        # "Channel 3"
        # "Channel 0"
        # "Set the X Axis to Autoscale"
        n48 = property on="Channel 0 Chart" class="WFChart (strict)"("XScale.ScaleFit"=u8 2 ("X Scale.Scale Fit")) -> ()  [unwired: 2 in, 2 out]
        n49 = property on="Channel 1 Chart" class="WFChart (strict)"("XScale.ScaleFit"=u8 2 ("X Scale.Scale Fit")) -> ()  [unwired: 2 in, 2 out]
        n50 = property on="Overview Chart" class="WFChart (strict)"("XScale.ScaleFit"=u8 2 ("X Scale.Scale Fit")) -> ()  [unwired: 2 in, 2 out]
        n51 = property on="Channel 2 Chart" class="WFChart (strict)"("XScale.ScaleFit"=u8 2 ("X Scale.Scale Fit")) -> ()  [unwired: 2 in, 2 out]
        n52 = property on="Channel 3 Chart" class="WFChart (strict)"("XScale.ScaleFit"=u8 2 ("X Scale.Scale Fit")) -> ()  [unwired: 2 in, 2 out]
        n53 = Increment(x=w233) -> (x+1=w227:i32)
        "Iterations Recorded" <- w227
        n54 = Divide(x=w222, y=10) -> (x/y=w230:dbl)
        n55 = Greater Or Equal?(x=w227, y=w232) -> (x >= y?=w228:bool)
        n56 = Reciprocal(x=w222) -> (1/x=w226:dbl)
        n57 = call-poly <vilib>:"DAQmxBase Read.vi"("task/channels in"=w224, "number of samples per channel"=w230, "timeout"=100.0, "error in"=w223) -> ("data"=w196:dbl[][])  [unwired: 9 in, 2 out]
        n58 = case shown="True" w200 {
          tunnel: w199 -> [_ w263]
          tunnel: w196 -> [_ w261]
          tunnel: [refnum<k34> refnum ("tdms file out") w259] -> w194
          frame False {
          }
          frame True {
            n59 = Index Array(array=w261, index (row)=0 ("index")) -> (element=w260:dbl[])  [unwired: 1 in]
            n60 = TDMS Write(0:w263, 7:string[] ["Channel 4"] ("channel name(s) in (Untitled)"), 9:w260) -> (4:w259:refnum<k34>)  [unwired: 3 in, 3 out]
          }
        }
        n61 = case shown="True" w190 {
          tunnel: w198 -> [_ w253]
          tunnel: w196 -> [_ w255]
          tunnel: [refnum<k34> refnum ("tdms file out") w254] -> w193
          frame False {
          }
          frame True {
            n62 = Index Array(array=w255, index (row)=1 ("index")) -> (element=w252:dbl[])  [unwired: 1 in]
            n63 = TDMS Write(0:w253, 7:string[] ["Channel 1"] ("channel name(s) in (Untitled)"), 9:w252) -> (4:w254:refnum<k34>)  [unwired: 3 in, 3 out]
          }
        }
        n64 = Multiply(x=20 ("y"), y=w226) -> (x*y=w201:dbl)
        n65 = case shown="True" w189 {
          tunnel: w197 -> [_ w249]
          tunnel: w196 -> [_ w247]
          tunnel: [refnum<k34> refnum ("tdms file out") w245] -> w192
          frame False {
          }
          frame True {
            n66 = Index Array(array=w247, index (row)=2 ("index")) -> (element=w246:dbl[])  [unwired: 1 in]
            n67 = TDMS Write(0:w249, 7:string[] ["Channel 2"] ("channel name(s) in (Untitled)"), 9:w246) -> (4:w245:refnum<k34>)  [unwired: 3 in, 3 out]
          }
        }
        n68 = Bundle("data"=w196, w202, 2, w213, w201, "Use Channel 2"=w189) -> (w215:T7)  [unwired: 1 in]
        n69 = Bundle("data"=w196, w202, 1, w213, w201, "Use Channel 1"=w190) -> (w216:T8)  [unwired: 1 in]
        n70 = Bundle("data"=w196, w202, 0, 20, w201, "Use Channel 0"=w200) -> (w218:T9)  [unwired: 1 in]
        n71 = Bundle("data"=w196, w202, 3, w213, w201, "Use Channel 3"=w188) -> (w212:T10)  [unwired: 1 in]
        n72 = call "Waveform Generation.vi"("Cluster"=w215) -> ("Output Y Values"=w184:dbl[], "Waveform"=w207:waveform(dbl))  [unwired: 9 in]
        n73 = call "Waveform Generation.vi"("Cluster"=w216) -> ("Output Y Values"=w185:dbl[], "Waveform"=w206:waveform(dbl))  [unwired: 9 in]
        n74 = call "Waveform Generation.vi"("Cluster"=w218) -> ("Output Y Values"=w186:dbl[], "Waveform"=w204:waveform(dbl))  [unwired: 9 in]
        n75 = call "Waveform Generation.vi"("Cluster"=w212) -> ("Output Y Values"=w183:dbl[], "Waveform"=w205:waveform(dbl))  [unwired: 9 in]
        n76 = case shown="True" w188 {
          tunnel: w195 -> [_ w242]
          tunnel: w196 -> [_ w240]
          tunnel: [refnum<k34> refnum ("tdms file out") w238] -> w191
          frame False {
          }
          frame True {
            n77 = Index Array(array=w240, index (row)=0 ("index")) -> (element=w239:dbl[])  [unwired: 1 in]
            n78 = TDMS Write(0:w242, 7:string[] ["Channel 3"] ("channel name(s) in (Untitled)"), 9:w239) -> (4:w238:refnum<k34>)  [unwired: 3 in, 3 out]
          }
        }
        n79 = Build Array(w186, w185, w184, w183) -> (w182:dbl[][])
        n80 = case shown="True" w228 {
          tunnel: [Enum_State_Typedef."Record" ("State") Enum_State_Typedef."Stop" ("State")] -> w229
          frame False {
            # "Continue recording"
          }
          frame True {
            # "Finished recording"
            n81 = One Button Dialog(message="Recording is Finished") -> ()  [unwired: 1 in, 1 out]
          }
        }
      }
      frame "Clear Display" {
        w273 = waveform(dbl) {"t0"=timestamp(0 s since 1904-01-01), "dt"=1.0, "Y"=[]} ("Waveform")
        (unwired) dbl[][] []
        w274 = waveform(dbl)[] [] ("History Data")
        # "clears the data"
        # "Clears the graph"
        # "Clears the chart history"
        # "This clears the chart display"
        n82 = property on="Overview Chart" class="WFChart (strict)"("History Data"=waveform(dbl)[][] []) -> ()  [unwired: 2 in, 2 out]
        n83 = property on="Channel 0 Chart" class="WFChart (strict)"("History Data"=w274) -> ()  [unwired: 2 in, 2 out]
        n84 = property on="Channel 2 Chart" class="WFChart (strict)"("History Data"=w274) -> ()  [unwired: 2 in, 2 out]
        n85 = property on="Channel 1 Chart" class="WFChart (strict)"("History Data"=w274) -> ()  [unwired: 2 in, 2 out]
        n86 = property on="Channel 3 Chart" class="WFChart (strict)"("History Data"=w274) -> ()  [unwired: 2 in, 2 out]
      }
      frame "Preview Data" {
        # "This is not incrementing"
        # "Turns off the X auto scale"
        n87 = property on="Overview Chart" class="WFChart (strict)"("XScale.Maximum"=w293) -> ()  [unwired: 2 in, 2 out]
        n88 = property on="Channel 2 Chart" class="WFChart (strict)"("XScale.Maximum"=w293) -> ()  [unwired: 2 in, 2 out]
        n89 = property on="Channel 3 Chart" class="WFChart (strict)"("XScale.Maximum"=w293) -> ()  [unwired: 2 in, 2 out]
        n90 = property on="Channel 1 Chart" class="WFChart (strict)"("XScale.Maximum"=w293) -> ()  [unwired: 2 in, 2 out]
        n91 = property on="Channel 0 Chart" class="WFChart (strict)"("XScale.ScaleFit"=u8 0 ("X Scale.Scale Fit")) -> ()  [unwired: 2 in, 2 out]
        n92 = property on="Overview Chart" class="WFChart (strict)"("XScale.ScaleFit"=u8 0 ("X Scale.Scale Fit")) -> ()  [unwired: 2 in, 2 out]
        n93 = property on="Channel 3 Chart" class="WFChart (strict)"("XScale.ScaleFit"=u8 0 ("X Scale.Scale Fit")) -> ()  [unwired: 2 in, 2 out]
        n94 = property on="Channel 1 Chart" class="WFChart (strict)"("XScale.ScaleFit"=u8 0 ("X Scale.Scale Fit")) -> ()  [unwired: 2 in, 2 out]
        n95 = property on="Channel 0 Chart" class="WFChart (strict)"("XScale.Maximum"=w293) -> ()  [unwired: 2 in, 2 out]
        n96 = Divide(x=w317, y=10) -> (x/y=w328:dbl)
        n97 = property on="Channel 2 Chart" class="WFChart (strict)"("XScale.ScaleFit"=u8 0 ("X Scale.Scale Fit")) -> ()  [unwired: 2 in, 2 out]
        n98 = call-poly <vilib>:"DAQmxBase Read.vi"("task/channels in"=w321, "number of samples per channel"=w328, "timeout"=100.0, "error in"=w320) -> ("data"=w297:dbl[][])  [unwired: 9 in, 2 out]
        n99 = Reciprocal(x=w317) -> (1/x=w327:dbl)
        n100 = Index Array(array=w292, index (row)=0) -> (element=w319:dbl[])  [unwired: 1 in]
        n101 = call "Preview Waveform.vi"("Decimation Multiple"=u16 20, "Channel #"=i8 2, "In Use?"=w296, "New Y Values"=w297, "Old Y Values"=w292) -> ("Output Y Values"=w284:dbl[])  [unwired: 6 in]
        n102 = Array Size(array=w319) -> (size(s)=w324:i32)
        n103 = call "Preview Waveform.vi"("Decimation Multiple"=u16 20, "Channel #"=i8 0, "In Use?"=w303, "New Y Values"=w297, "Old Y Values"=w292) -> ("Output Y Values"=w286:dbl[])  [unwired: 6 in]
        n104 = call "Preview Waveform.vi"("Decimation Multiple"=u16 20, "Channel #"=i8 1, "In Use?"=w299, "New Y Values"=w297, "Old Y Values"=w292) -> ("Output Y Values"=w285:dbl[])  [unwired: 6 in]
        n105 = call "Preview Waveform.vi"("Decimation Multiple"=u16 20, "Channel #"=i8 3, "In Use?"=w306, "New Y Values"=w297, "Old Y Values"=w292) -> ("Output Y Values"=w283:dbl[])  [unwired: 6 in]
        n106 = Multiply(x=20 ("y"), y=w327) -> (x*y=w316:dbl)
        n107 = Multiply(x=w324, y=w316) -> (x*y=w323:dbl)
        n108 = Bundle By Name("Y"=w284, "dt"=w316) -> (w289:waveform(dbl))  [unwired: 1 in]
        n109 = Bundle By Name("Y"=w285, "dt"=w316) -> (w290:waveform(dbl))  [unwired: 1 in]
        n110 = Bundle By Name("Y"=w286, "dt"=w316) -> (w291:waveform(dbl))  [unwired: 1 in]
        n111 = Bundle By Name("Y"=w283, "dt"=w316) -> (w288:waveform(dbl))  [unwired: 1 in]
        n112 = Less?(x=w323, y=w293) -> (x < y?=w318:bool)
        n113 = Build Array(w286, w285, w284, w283) -> (w282:dbl[][])
        n114 = Build Array(w291, w290, w289, w288) -> (w287:waveform(dbl)[])
        n115 = case shown="False" w318 {
          tunnel: [Enum_State_Typedef."Prepreview Handling" ("State") Enum_State_Typedef."Preview Data" ("State")] -> w325
          frame False {
          }
          frame True {
          }
        }
      }
      frame "Create File" {
        # "This Creates and writes the header of the file with all the user inputted data"
        n116 = case shown="True" w351 {
          tunnel: [refnum<k34> refnum ("tdms file out") w388] -> w343
          frame False {
          }
          frame True {
            n117 = call "File Dialog"("prompt"="Select or Create a File for Channel 3") -> ("selected path"=w392:path)  [unwired: 11 in, 3 out]
            n118 = TDMS Open(10:T5."create" ("operation (0:open)"), 11:w392) -> (3:w389:refnum<k34>)  [unwired: 5 in, 1 out]
            n119 = call "Header Data Creator.vi"("tdms file in"=w389, "Amplifier Metadata"="Amplifier Channel 0", "User Data"="User Data Channel 0") -> ("tdms file out"=w388:refnum<k34>)  [unwired: 6 in, 1 out]
          }
        }
        n120 = Enqueue Element(queue=w360, element=Enum_State_Typedef."Record", error in (no error)=w359) -> ()  [unwired: 1 in, 3 out]
        n121 = case shown="True" w350 {
          tunnel: [refnum<k34> refnum ("tdms file out") w378] -> w342
          frame False {
          }
          frame True {
            n122 = call "File Dialog2"("prompt"="Select or Create a File for Channel 2") -> ("selected path"=w383:path)  [unwired: 11 in, 3 out]
            n123 = TDMS Open(10:T5."create" ("operation (0:open)"), 11:w383) -> (3:w381:refnum<k34>)  [unwired: 5 in, 1 out]
            n124 = call "Header Data Creator.vi"("tdms file in"=w381, "Amplifier Metadata"="Amplifier Channel 1", "User Data"="User Data Channel 1") -> ("tdms file out"=w378:refnum<k34>)  [unwired: 6 in, 1 out]
          }
        }
        n125 = Get Date/Time String(date format (0)=enum16{"short", "long", "abbreviated"}."short") -> (date string=→"Date mm/dd/yy":string, time string=→"Start Time hr/min":string)  [unwired: 2 in]
        n126 = case shown="True" w349 {
          tunnel: [refnum<k34> refnum ("tdms file out") w370] -> w341
          frame False {
          }
          frame True {
            n127 = call "File Dialog3"("prompt"="Select or Create a File for Channel 1") -> ("selected path"=w375:path)  [unwired: 11 in, 3 out]
            n128 = TDMS Open(10:T5."create" ("operation (0:open)"), 11:w375) -> (3:w371:refnum<k34>)  [unwired: 5 in, 1 out]
            n129 = call "Header Data Creator.vi"("tdms file in"=w371, "Amplifier Metadata"="Amplifier Channel 2", "User Data"="User Data Channel 2") -> ("tdms file out"=w370:refnum<k34>)  [unwired: 6 in, 1 out]
          }
        }
        n130 = case shown="True" w348 {
          tunnel: [refnum<k34> refnum ("tdms file out") w364] -> w340
          frame False {
          }
          frame True {
            n131 = call "File Dialog4"("prompt"="Select or Create a File for Channel 0") -> ("selected path"=w367:path)  [unwired: 11 in, 3 out]
            n132 = TDMS Open(10:T5."create" ("operation (0:open)"), 11:w367) -> (3:w365:refnum<k34>)  [unwired: 5 in, 1 out]
            n133 = call "Header Data Creator.vi"("tdms file in"=w365, "Amplifier Metadata"="Amplifier Channel 3", "User Data"="User Data Channel 3") -> ("tdms file out"=w364:refnum<k34>)  [unwired: 6 in, 1 out]
          }
        }
      }
      frame "Prepreview Handling" {
        (unwired) dbl[][] [] ("Output Y Values")
        w399 = waveform(dbl)[] [] ("History Data")
        w400 = waveform(dbl) {"t0"=timestamp(0 s since 1904-01-01), "dt"=1.0, "Y"=[]}
        # "This clears the Chart history"
        # "This clears the data before the preview data state starts"
        n134 = property on="Overview Chart" class="WFChart (strict)"("History Data"=waveform(dbl)[][] []) -> ()  [unwired: 2 in, 2 out]
        n135 = property on="Channel 2 Chart" class="WFChart (strict)"("History Data"=w399) -> ()  [unwired: 2 in, 2 out]
        n136 = property on="Channel 3 Chart" class="WFChart (strict)"("History Data"=w399) -> ()  [unwired: 2 in, 2 out]
        n137 = property on="Channel 1 Chart" class="WFChart (strict)"("History Data"=w399) -> ()  [unwired: 2 in, 2 out]
        n138 = property on="Channel 0 Chart" class="WFChart (strict)"("History Data"=w399) -> ()  [unwired: 2 in, 2 out]
      }
    }
    "Channel 0 Chart" <- w30
    "State" <- w44
    "Channel 1 Chart" <- w28
    "Channel 3 Chart" <- w29
    "Channel 2 Chart" <- w27
    "Overview Chart" <- w11
  }
  n139 = while {
    tunnel: w8 -> [w412]
    tunnel: w7 -> [w411]
    tunnel: w2 -> [w409]
    tunnel: w1 -> [w408]
    stop <- w410 stop-if-true
    # "Event Handling Loop"
    n140 = event shown="[3] \"Stop Preview\": Value Change" {
      selector: _ -> [_ _ _ _ _ _ _ _]
      dyn-events: _ -> [_ _ _ _ _ _ _ _]
      timeout: _ -> [_ _ _ _ _ _ _ _]
      tunnel: [FALSE ("Exit Button") "Exit Button" _ _ _ _ _ _] -> w410
      tunnel: w412 -> [_ w418 w424 w427 w430 w435 w440 w443]
      tunnel: w411 -> [_ w417 w423 w426 w429 w434 w439 w442]
      tunnel: [_ w416 w421 _ _ w432 w437 _] -> _
      tunnel: [_ w415 w420 _ _ w433 w438 _] -> _
      event Timeout {
        n141 = event-data() -> ()  [unwired: 1 in, 3 out]
      }
      event "Exit Button": Value Change {
        n142 = event-data() -> ()  [unwired: 1 in, 1 out]
        n143 = Enqueue Element(queue=w418, element=Enum_State_Typedef."Exit", error in (no error)=w417) -> (queue out=w416:refnum<queue>, error out=w415:errorcluster)  [unwired: 1 in, 1 out]
      }
      event "Preview Button": Value Change {
        n144 = event-data() -> ()  [unwired: 1 in, 6 out]
        n145 = Enqueue Element(queue=w424, element=Enum_State_Typedef."Preview Data", error in (no error)=w423) -> (queue out=w421:refnum<queue>, error out=w420:errorcluster)  [unwired: 1 in, 1 out]
      }
      event "Stop Preview": Value Change {
        n146 = event-data() -> ()  [unwired: 1 in, 6 out]
        n147 = Enqueue Element(queue=w427, element=Enum_State_Typedef."", error in (no error)=w426) -> ()  [unwired: 1 in, 3 out]
      }
      event "OK Button": Value Change {
        n148 = event-data() -> ()  [unwired: 1 in, 6 out]
        n149 = Enqueue Element(queue=w430, element=Enum_State_Typedef."Set the Sample Clock", error in (no error)=w429) -> ()  [unwired: 1 in, 3 out]
      }
      event "Stop Button": Value Change {
        n150 = event-data() -> ()  [unwired: 1 in, 6 out]
        n151 = Enqueue Element(queue=w435, element=Enum_State_Typedef."Stop", error in (no error)=w434) -> (queue out=w432:refnum<queue>, error out=w433:errorcluster)  [unwired: 1 in, 1 out]
      }
      event "Record Button": Value Change {
        n152 = event-data() -> ()  [unwired: 1 in, 6 out]
        n153 = Enqueue Element(queue=w440, element=Enum_State_Typedef."Create File", error in (no error)=w439) -> (queue out=w437:refnum<queue>, error out=w438:errorcluster)  [unwired: 1 in, 1 out]
      }
      event "Clear Display": Value Change {
        n154 = event-data() -> ()  [unwired: 1 in, 6 out]
        n155 = Enqueue Element(queue=w443, element=Enum_State_Typedef."Clear Display", error in (no error)=w442) -> ()  [unwired: 1 in, 3 out]
      }
    }
    n156 = Enqueue Element(queue=w409, element=w410, error in (no error)=w408) -> ()  [unwired: 1 in, 3 out]
  }
